vi "Configure Normalize.vi"(8 "error in (no error)":errorcluster, 9 "Normalized Reference Level (0 dB)":dbl format="%.0g", 10 "Enable Normalize (F: Disable)":bool, 11 "VISA resource name":refnum<visa-resource-name>) -> (0 "error out":errorcluster, 3 "VISA resource name out":refnum<visa-resource-name>)   [LabVIEW 2014, in "Agilent MXA Series.lvlib"]
doc: "Configures the normalize function. On each sweep, the normalized trace (Trace 3) is subtracted from Trace 1 and the result is added to the normalized reference level. This arithmetic assumes all values are in decibel\nunits.\n\n<B>Note:</B>\nYou can use this VI only under Swept SA measurement type."
uses:
  Agilent MXA Series.lvlib
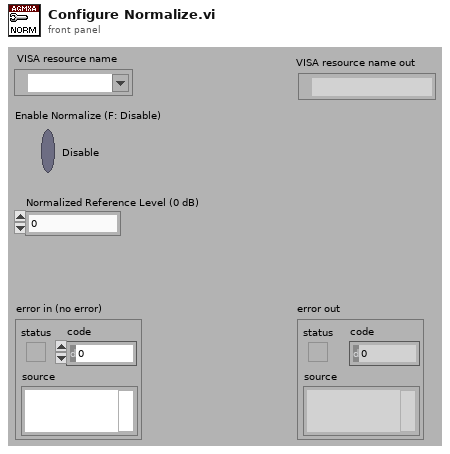
[diagram p1: front panel]
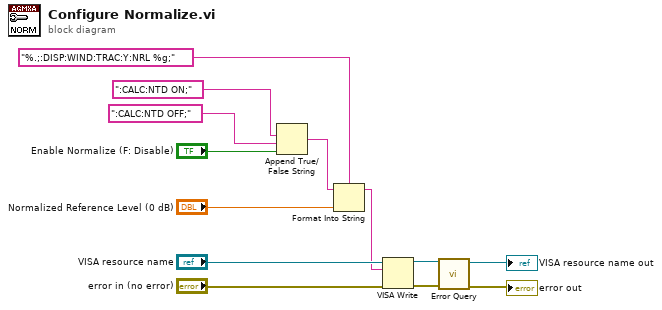
[diagram p0: block diagram]
diagram:
  n1 = Append True/False String(1:"Enable Normalize (F: Disable)", 2:":CALC:NTD OFF;" ("true string"), 3:":CALC:NTD ON;" ("true string")) -> (0:w8:string)  [unwired: 1 in]
  n2 = Format Into String(format string="%.;:DISP:WIND:TRAC:Y:NRL %g;", initial string=w8, "Normalized Reference Level (0 dB)") -> (resulting string=w5:string)  [unwired: 1 in, 1 out]
  n3 = VISA Write(VISA resource name="VISA resource name", write buffer=w5, error in (no error)="error in (no error)") -> (VISA resource name out=w4:refnum<visa-resource-name>, error out=w3:errorcluster)  [unwired: 1 out]
  n4 = call "Error Query.vi"("error in (no error)"=w3, "VISA resource name"=w4) -> ("error out"=→"error out":errorcluster, "VISA resource name out"=→"VISA resource name out":refnum<visa-resource-name>)  [unwired: 6 in, 2 out]
